vi "Configure.vi"(8 "error in (no error)":errorcluster, 10 "ID":string, 11 "MKS999 in":refnum<class "MKS999.lvclass">) -> (0 "error out":errorcluster, 3 "MKS999 out":refnum<class "MKS999.lvclass">)   [LabVIEW 2016, in "MKS999.lvlib" / "MKS999.lvclass"]
uses:
  MKS999.lvclass
  MKS999.lvclass/MKS999.ctl
  <vilib>/Utility/config.llb/Read Key (U32).vi
  <vilib>/Utility/config.llb/Read Key (String).vi
  <vilib>/Utility/config.llb/NI_LVConfig.lvlib
panel:
  in  "error in (no error) 2":errorcluster
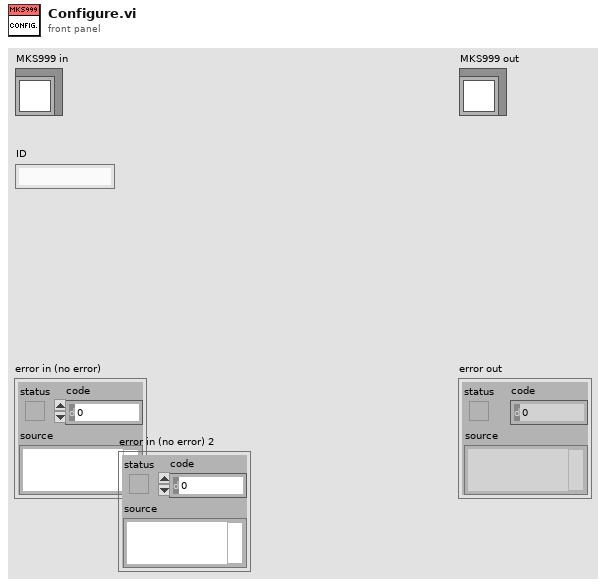
[diagram p1: front panel]
types:
  T1 = typedef "NI_LVConfig.lvlib/Config Data RefNum.ctl" = refnum<k1>
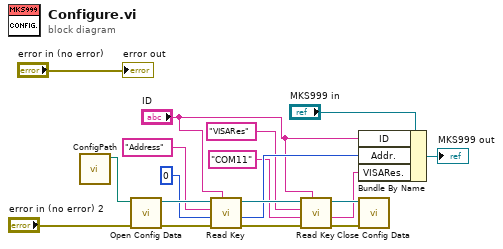
[diagram p0: block diagram]
diagram:
  n1 = call "ConfigPath.vi"() -> ("ConfigPath"=w17:path)  [unwired: 11 in]
  n2 = call <vilib>:"Open Config Data.vi"("error in (no error)"="error in (no error) 2", "configuration file path"=w17) -> ("error out"=w14:errorcluster, "refnum"=w16:T1)  [unwired: 7 in, 1 out]
  n3 = call-poly <vilib>:"Read Key.vi"("section"="ID", "error in (no error)"=w14, "default value"=u8 0, "key"="Address", "refnum"=w16) -> ("error out"=w12:errorcluster, "value"=w8:u32, "refnum out"=w13:T1)  [unwired: 3 in, 1 out]
  n4 = call-poly <vilib>:"Read Key.vi"("section"="ID", "error in (no error)"=w12, "default value"="COM11" ("key"), "key"="VISARes", "refnum"=w13) -> ("error out"=w10:errorcluster, "value"=w5:string, "refnum out"=w11:T1)  [unwired: 3 in, 1 out]
  n5 = Bundle By Name(cluster="MKS999 in", "ID"="ID", "Addr."=w8, "VISARes."=w5) -> (→"MKS999 out":refnum<class "MKS999.lvclass">)
  n6 = call <vilib>:"Close Config Data.vi"("error in (no error)"=w10, "refnum"=w11) -> ()  [unwired: 8 in, 2 out]
  "error out" <- "error in (no error)"
